vi "Test shm issue Command start LV.vi"(8 "error in (no error)":errorcluster, 11 "command_start_Ctl":cluster{"size":i32, "data":string}) -> (0 "error out":errorcluster, 2 "function return":i32, 3 "command_start_Ctl out":cluster{"size":i32, "data":string})   [LabVIEW 2018, in "SALLV_Test.lvlib"]
doc: "int Test_shm_issueCommand_startLV(Test_command_startLV *command_start_Ctl );"
uses:
  SALLV_Test.lvlib
  SALLV_Test.so
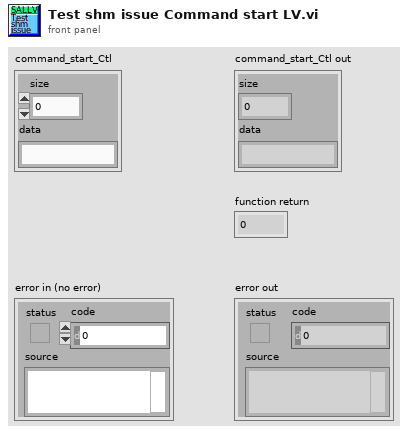
[diagram p1: front panel]
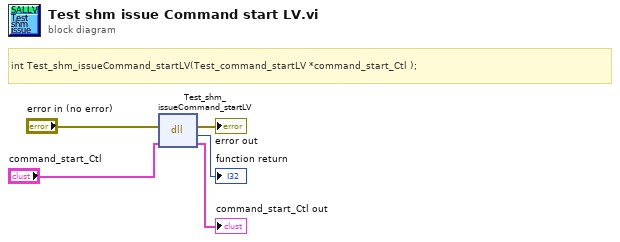
[diagram p0: block diagram]
diagram:
  # "int Test_shm_issueCommand_startLV(Test_command_startLV *command_start_Ctl );"
  n1 = dll-call lib="home/ttsai/Documents/salLabVIEWtestData/SALLV_Test.*" fn="Test_shm_issueCommand_startLV"(error in="error in (no error)", "command_start_Ctl"="command_start_Ctl") -> (error out=→"error out":errorcluster, →"function return":i32, "command_start_Ctl"=→"command_start_Ctl out":cluster{"size":i32, "data":string})  [unwired: 2 in, 1 out]
